vi "Add Embedded Data Logger Custom Device.vi"(8 "error in":errorcluster, 10 "name":string="Embedded Data Logger", 11 "target in":refnum<k39>) -> (0 "error out":errorcluster, 2 "embedded data logger":T1 format="%.0x", 3 "target out":refnum<k39>)   [LabVIEW 2027, in "Embedded Data Logger Scripting.lvlib"]
uses:
  Embedded Data Logger Scripting.lvlib
  C:/NetCore/niveristand-embedded-data-logger-custom-device/Source/Scripting/Custom Device/Add Embedded Data Logger Custom Device.vi/NationalInstruments.VeriStand.SystemDefinitionAPI
  NationalInstruments.VeriStand.SystemDefinitionAPI
  Shared/Constants.vi
  Shared/Embedded Data Logger Shared.lvlib
  <vilib>/NI VeriStand/Custom Device Tools/Custom Device Utility Library/Custom Device Utility Library.lvlib
  <vilib>/NI VeriStand/Custom Device API/Custom Device Item Ref.ctl
  <vilib>/NI VeriStand/Custom Device API/Custom Device API.lvlib
  C:/NetCoreDLL/NationalInstruments.VeriStand.SystemDefinitionAPI.dll
  NetCoreDLL/NationalInstruments.VeriStand.SystemDefinitionAPI.dll
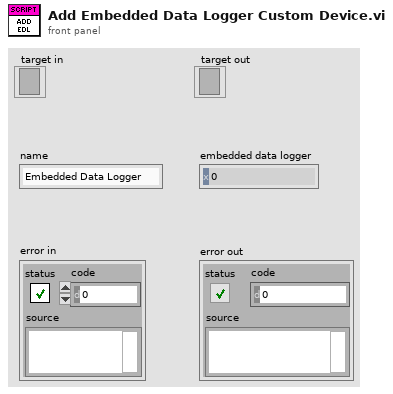
[diagram p1: front panel]
types:
  T1 = typedef "Custom Device API.lvlib/Custom Device Item Ref.ctl" = u64
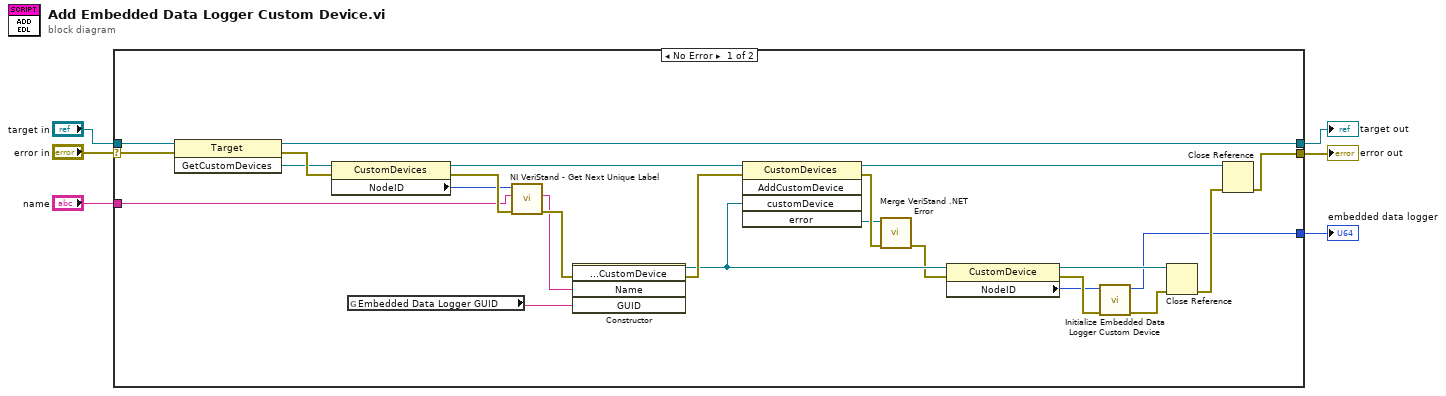
[diagram p0: block diagram]
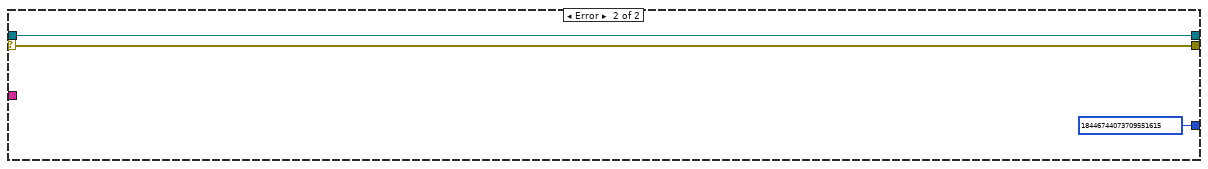
[diagram p2: hidden frame]
diagram:
  n1 = case shown="No Error" "error in" {
    selector: "error in" -> [w28 w34]
    tunnel: "target in" -> [w27 w33]
    tunnel: "name" -> [w24 _]
    tunnel: [w18 w33] -> w2
    tunnel: [w10 w34] -> w3
    tunnel: [w7 T1 18446744073709551615 ("embedded data logger out")] -> w1
    frame No Error {
      n2 = invoke class="Target" method="GetCustomDevices"(reference=w27, error in=w28) -> (reference out=w18:refnum<k39>, error out=w30:errorcluster, "GetCustomDevices"=w29:refnum<k39>)  [unwired: 1 in]
      n3 = property class="CustomDevices"(reference=w29, error in=w30) -> (reference out=w20:refnum<k39>, error out=w26:errorcluster, "NodeID"=w25:u64)
      n4 = global read "Constants.vi" "Embedded Data Logger GUID"() -> (w21:string)
      n5 = call <vilib>:"NI VeriStand - Get Next Unique Label.vi"("error in (no error)"=w26, "Label"=w24, "Parent Ref in"=w25) -> ("error out"=w23:errorcluster, "Label out"=w22:string)  [unwired: 5 in, 2 out]
      n6 = constructor class="CustomDevice"(error in=w23, "Name"=w22, "GUID"=w21) -> (reference out=w16:refnum<k39>, error out=w19:errorcluster)  [unwired: 2 in, 3 out]
      n7 = invoke class="CustomDevices" method="AddCustomDevice"(reference=w20, error in=w19, "customDevice"=w16) -> (reference out=w17:refnum<k39>, error out=w31:errorcluster, "error"=w9:refnum<k39>)  [unwired: 2 in, 2 out]
      n8 = call "Merge VeriStand .NET Error.vi"("error in"=w31, "NationalInstruments.VeriStand.Error"=w9) -> ("error out"=w8:errorcluster)  [unwired: 9 in]
      n9 = property class="CustomDevice"(reference=w16, error in=w8) -> (reference out=w14:refnum<k39>, error out=w13:errorcluster, "NodeID"=w12:u64)
      n10 = call "Initialize Embedded Data Logger Custom Device.vi"("error in"=w13, "embedded data logger in"=w12) -> ("error out"=w11:errorcluster, "embedded data logger out"=w7:T1)  [unwired: 8 in]
      n11 = Close Reference(reference=w14, error in (no error)=w11) -> (error out=w15:errorcluster)
      n12 = Close Reference(reference=w17, error in (no error)=w15) -> (error out=w10:errorcluster)
    }
    frame Error {
    }
  }
  "target out" <- w2
  "error out" <- w3
  "embedded data logger" <- w1
